vi "ParseArguments.vi"(8 "error in (no error)":errorcluster, 10 "Inputs":string[](array[string]), 11 "RunVIAnalyzer in":refnum<class "RunVIAnalyzer.lvclass">) -> (0 "error out":errorcluster, 3 "RunVIAnalyzer out":refnum<class "RunVIAnalyzer.lvclass">)   [LabVIEW 2014, in "RunVIAnalyzer.lvclass"]
uses:
  RunVIAnalyzer.lvclass
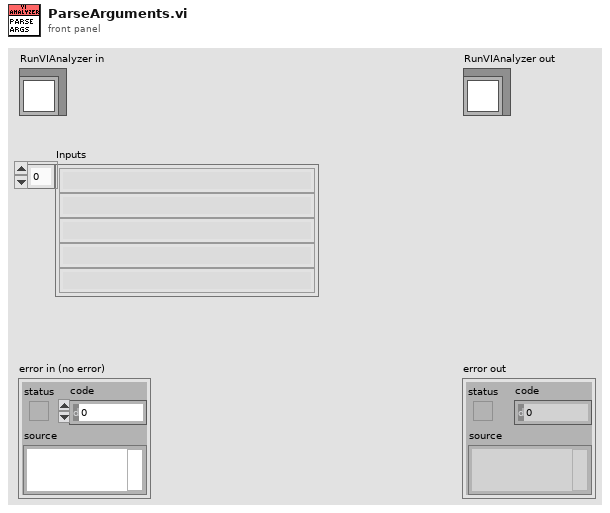
[diagram p1: front panel]
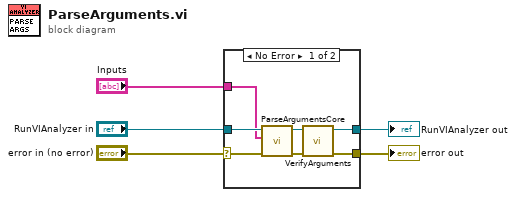
[diagram p0: block diagram]
diagram:
  n1 = case shown="No Error" "error in (no error)" {
    selector: "error in (no error)" -> [w10 w14]
    tunnel: [w8 w14] -> w4
    tunnel: [w6 w13] -> w3
    tunnel: "RunVIAnalyzer in" -> [w12 w13]
    tunnel: "Inputs" -> [w11 _]
    frame No Error {
      n2 = call "ParseArgumentsCore.vi"("error in (no error)"=w10, "Inputs"=w11, "RunVIAnalyzer in"=w12) -> ("error out"=w9:errorcluster, "RunVIAnalyzer out"=w7:refnum<class "RunVIAnalyzer.lvclass">)  [unwired: 7 in]
      n3 = call "VerifyArguments.vi"("error in (no error)"=w9, "RunVIAnalyzer in"=w7) -> ("error out"=w8:errorcluster, "RunVIAnalyzer out"=w6:refnum<class "RunVIAnalyzer.lvclass">)  [unwired: 8 in]
    }
    frame Error {
    }
  }
  "error out" <- w4
  "RunVIAnalyzer out" <- w3
